vi "Post Error.vi"(0 "Web App Handle In":T1, 2 "message":string, 3 "error in":errorcluster) -> (7 "Web App Handle Out":T1, 8 "response":string, 10 "error out":errorcluster)   [LabVIEW 2013, in "Web Messaging API.lvlib"]
doc: "Posts an error to the Web Messaging service, more information can be found at https://myrio.niwsc.com"
uses:
  Web Messaging API.lvlib
  Web Messaging Handle.ctl
  <vilib>/Utility/error.llb/DialogType.ctl
  <vilib>/httpClient/POSTBuffer.vi
  <vilib>/httpClient/LabVIEWHTTPClient.lvlib
panel:
  in  "Error Object":T2={"type"="labview_error", "field_status"=FALSE, "body"={"und"=[{"value"=" "}]}, "field_source"={"und"=[{"value"=" "}]}, "field_code"={"und"=[{"value"=0}]}}
  out "JSON Object":string
  out "headers":string
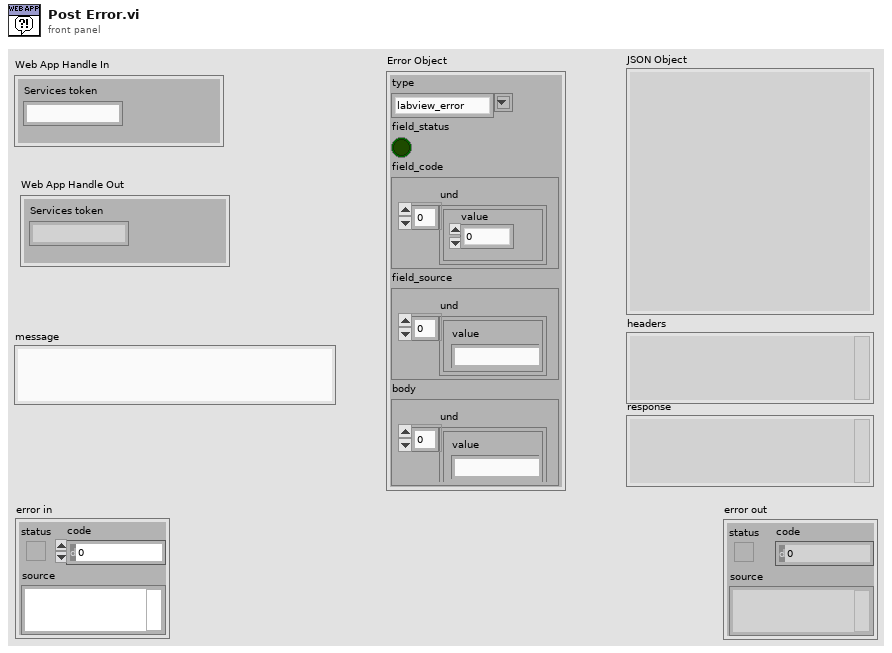
[diagram p1: front panel]
types:
  T1 = typedef "Web Messaging API.lvlib/Web Messaging Handle.ctl" = cluster{"Services token":string}
  T2 = cluster{"type":string, "field_status":bool, "body":cluster{"und":cluster{"value":string}[]}, "field_source":cluster{"und":cluster{"value":string}[]}, "field_code":cluster{"und":cluster{"value":i32}[]}}
  T3 = typedef "DialogType.ctl" = u16
  T4 = typedef "LabVIEWHTTPClient.lvlib/ClientHandle.ctl" = refnum<k1>
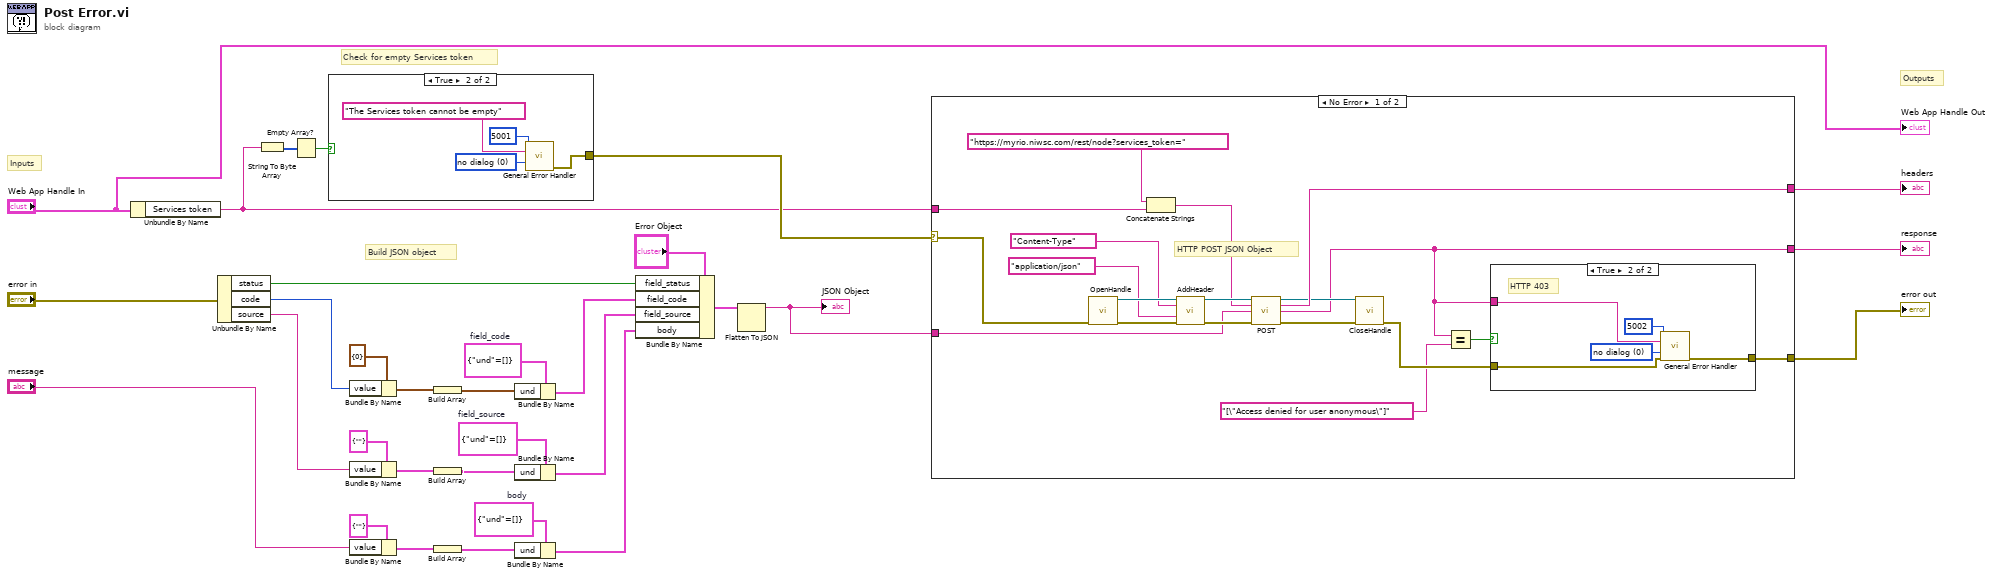
[diagram p0: block diagram]
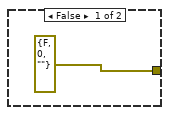
[diagram p2: hidden frame]
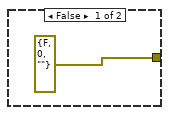
[diagram p4: hidden frame]
diagram:
  w8 = cluster{"und":cluster{"value":string}[]} {"und"=[]}  # field_source
  w11 = cluster{"und":cluster{"value":i32}[]} {"und"=[]}  # field_code
  w16 = cluster{"und":cluster{"value":string}[]} {"und"=[]}  # body
  # "Check for empty Services token"
  # "Build JSON object"
  # "Outputs"
  # "Inputs"
  n1 = Unbundle By Name("Web App Handle In") -> ("Services token"=w2:string)
  n2 = Unbundle By Name("error in") -> ("status"=w24:bool, "code"=w9:i32, "source"=w22:string)
  n3 = String To Byte Array(string=w2) -> (unsigned byte array=w5:u8[])
  n4 = Empty Array?(array=w5) -> (empty?=w4:bool)
  n5 = case shown="True" w4 {
    tunnel: [errorcluster {"status"=FALSE, "code"=0, "source"=""} ("error out") w34] -> w3
    frame False {
    }
    frame True {
      w35 = T3 0 items=["no dialog", "OK message", "continue or stop message", "OK message + warnings", "continue/stop + warnings"] ("type of dialog (OK msg:1)")
      n6 = call <vilib>:"General Error Handler.vi"("[error code] (0)"=5001, "[error source] (\" \")"="The Services token cannot be empty" ("[error source] (\" \")"), "type of dialog (OK msg:1)"=w35) -> ("error out"=w34:errorcluster)  [unwired: 8 in, 4 out]
    }
  }
  n7 = Bundle By Name(cluster=cluster{"value":i32} {"value"=0} ("Cluster"), "value"=w9) -> (w14:cluster{"value":i32})
  n8 = Bundle By Name(cluster=cluster{"value":string} {"value"=""} ("Cluster"), "value"=w22) -> (w21:cluster{"value":string})
  n9 = Bundle By Name(cluster=cluster{"value":string} {"value"=""} ("Cluster"), "value"="message") -> (w19:cluster{"value":string})
  n10 = Build Array(w14) -> (w13:cluster{"value":i32}[])
  n11 = Build Array(w21) -> (w7:cluster{"value":string}[])
  n12 = Build Array(w19) -> (w17:cluster{"value":string}[])
  n13 = Bundle By Name(cluster=w11, "und"=w13) -> (w12:cluster{"und":cluster{"value":i32}[]})
  n14 = Bundle By Name(cluster=w8, "und"=w7) -> (w20:cluster{"und":cluster{"value":string}[]})
  n15 = Bundle By Name(cluster=w16, "und"=w17) -> (w15:cluster{"und":cluster{"value":string}[]})
  n16 = Bundle By Name(cluster="Error Object", "field_status"=w24, "field_code"=w12, "field_source"=w20, "body"=w15) -> (w23:T2)
  n17 = Flatten To JSON(anything=w23) -> (JSON string=w26:string)  [unwired: 2 in, 1 out]
  "JSON Object" <- w26
  n18 = case shown="No Error" w3 {
    selector: w3 -> [w42 w62]
    tunnel: w2 -> [w55 _]
    tunnel: [w54 _] -> w31
    tunnel: [w37 _] -> w30
    tunnel: [w40 w62] -> w28
    tunnel: w26 -> [w43 _]
    frame No Error {
      # "HTTP POST JSON Object"
      n19 = call <vilib>:"OpenHandle.vi"("error in (no error)"=w42) -> ("client handle out"=w51:T4, "error out"=w50:errorcluster)  [unwired: 13 in]
      n20 = Concatenate Strings("https://myrio.niwsc.com/rest/node?services_token=" ("value"), w55) -> (w44:string)
      n21 = call <vilib>:"AddHeader.vi"("client handle"=w51, "header"="Content-Type", "value"="application/json", "error in (no error)"=w50) -> ("client handle out"=w46:T4, "error out"=w47:errorcluster)  [unwired: 10 in]
      n22 = call-poly <vilib>:"POST.vi"("client handle"=w46, "url"=w44, "buffer"=w43, "error in (no error)"=w47) -> ("client handle out"=w52:T4, "headers"=w54:string, "body"=w37:string, "error out"=w53:errorcluster)  [unwired: 8 in]
      n23 = call <vilib>:"CloseHandle.vi"("client handle"=w52, "error in (no error)"=w53) -> ("error out"=w41:errorcluster)  [unwired: 13 in]
      n24 = Equal?(x=w37, y="[\"Access denied for user anonymous\"]") -> (x = y?=w38:bool)
      n25 = case shown="True" w38 {
        tunnel: [errorcluster {"status"=FALSE, "code"=0, "source"=""} ("error out") w60] -> w40
        tunnel: w41 -> [_ w58]
        tunnel: w37 -> [_ w57]
        frame False {
        }
        frame True {
          w61 = T3 0 items=["no dialog", "OK message", "continue or stop message", "OK message + warnings", "continue/stop + warnings"] ("type of dialog (OK msg:1)")
          # "HTTP 403"
          n26 = call <vilib>:"General Error Handler.vi"("[error code] (0)"=5002, "[error source] (\" \")"=w57, "type of dialog (OK msg:1)"=w61, "error in (no error)"=w58) -> ("error out"=w60:errorcluster)  [unwired: 7 in, 4 out]
        }
      }
    }
    frame Error {
    }
  }
  "headers" <- w31
  "response" <- w30
  "error out" <- w28
  "Web App Handle Out" <- "Web App Handle In"
